vi "SDCP SMF Receiver and Transmitter - View Trace Data.vi"() -> ()   [LabVIEW 2020]
panel:
  in  "Parameter Excel File Path":path=path "E:/Projects/System Diagnostics and Control Protocol/SDCP_LabVIEW/Parameter Files/Motion Processing Board - Standard Message Frame List.csv"
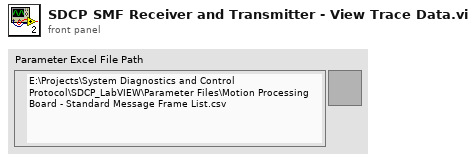
[diagram p1: front panel]
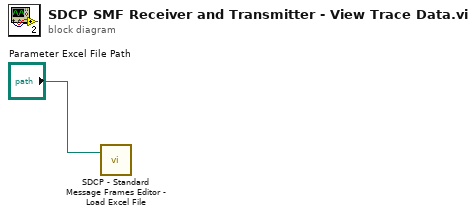
[diagram p0: block diagram]
diagram:
  n1 = call "SDCP - Standard Message Frames Editor - Load Excel File.vi"("Excel File Path"="Parameter Excel File Path") -> ()  [unwired: 1 in, 2 out]
